vi "Initialize Connection.vi"(8 "error in (no error)":errorcluster, 10 "Port":u16, 11 "IP Address":string) -> (0 "error out":errorcluster, 3 "NodeRed-LV-Interface out":refnum<class "NodeRed-LV-Interface.lvclass">)   [LabVIEW 2020, in "NodeRed-LV-Interface.lvclass"]
doc: "Initialize the connection between the Node-Red UDP connection to LabVIEW UDP Interface. IP Address and Port should be define based on the Node-Red Configuration."
uses:
  NodeRed-LV-Interface.lvclass
  NodeRed-LV-Interface.lvclass/NodeRed-LV-Interface.ctl
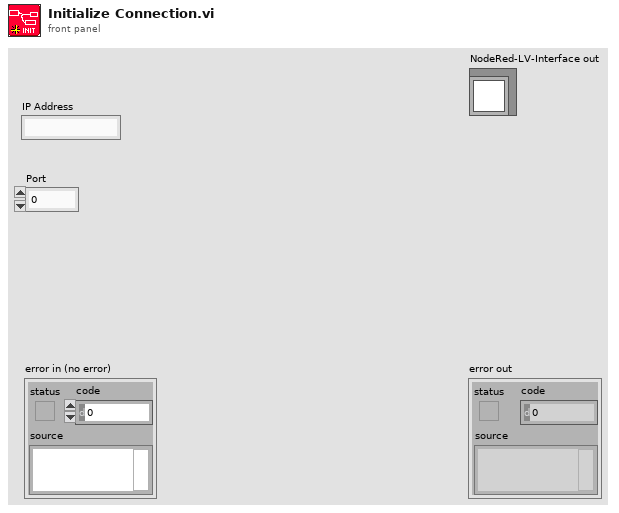
[diagram p1: front panel]
types:
  T1 = cluster{"Send data":refnum<user-event>, "Receive data":refnum<user-event>, "UDP Engine":refnum<vi>, "IP Address":string, "Port":u16}
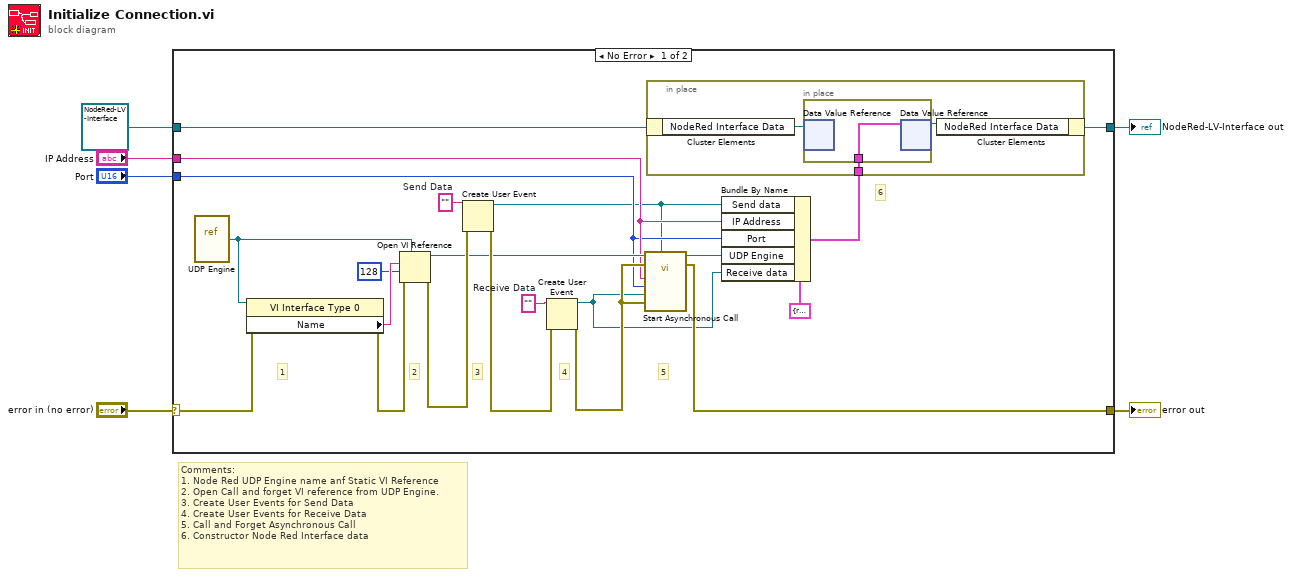
[diagram p0: block diagram]
diagram:
  # "Comments:\n1. Node Red UDP Engine name anf Static VI Reference\n2. Open Call and forget VI reference from UDP Engine.\n3. Create User Events for Send Data\n4. Create User Events for Receive Data\n5. Call and Forget Asynchronous Call\n6. Constructor Node Red Interface data"
  n1 = case shown="No Error" "error in (no error)" {
    selector: "error in (no error)" -> [w25 w33]
    tunnel: [w17 w33] -> w5
    tunnel: [w7 w32] -> w3
    tunnel: refnum<class "NodeRed-LV-Interface.lvclass"> refnum ("NodeRed-LV-Interface in") -> [w15 w32]
    tunnel: "IP Address" -> [w13 _]
    tunnel: "Port" -> [w12 _]
    frame No Error {
      w22 = ""  # Receive Data
      w23 = ""  # Send Data
      # "6"
      # "5"
      # "4"
      # "3"
      # "2"
      # "1"
      n2 = vi-ref "UDP Engine.vi"() -> (w26:refnum<vi>)
      n3 = property class="VI Interface Type 0"(reference=w26, error in=w25) -> (error out=w24:errorcluster, "Name"=w27:string)  [unwired: 1 out]
      n4 = Open VI Reference(type specifier VI Refnum (for type only)=w26, vi path=w27, options=128, error in (no error)=w24) -> (vi reference=w18:refnum<vi>, error out=w21:errorcluster)  [unwired: 2 in]
      n5 = Create User Event(user event datatype=w23, error in=w21) -> (user event=w11:refnum<user-event>, error out=w20:errorcluster)
      n6 = Create User Event(user event datatype=w22, error in=w20) -> (user event=w9:refnum<user-event>, error out=w16:errorcluster)
      n7 = call-by-ref "Start Asynchronous Call"(reference=w18, error in=w16, "Send data"=w11, 8:"error in (no error)"=w16, "Receive data"=w9, "Port"=w12, "IP Address"=w13) -> (reference out=w10:refnum<vi>, error out=w17:errorcluster)  [unwired: 6 in, 1 out]
      n8 = Bundle By Name(cluster=T1 {"Send data"=refnum, "Receive data"=refnum, "UDP Engine"=refnum, "IP Address"="", "Port"=0} ("data value"), "Send data"=w11, "IP Address"=w13, "Port"=w12, "UDP Engine"=w10, "Receive data"=w9) -> (w8:T1)
      n9 = in-place {
        in-place-border: w8 -> [w28]
        n10 = in-place-cluster #1(w15) -> ("NodeRed Interface Data"=w30:refnum<data-value>)
        n11 = in-place {
          in-place-border: w28 -> [w31]
          n12 = in-place-dvr #2(w30) -> ()  [unwired: 2 out]
          n13 = in-place-dvr #2(w31) -> (w29:refnum<data-value>)  [unwired: 1 out]
        }
        n14 = in-place-cluster #1("NodeRed Interface Data"=w29) -> (w7:refnum<class "NodeRed-LV-Interface.lvclass">)
      }
    }
    frame Error {
    }
  }
  "error out" <- w5
  "NodeRed-LV-Interface out" <- w3
